vi "19052_get_test_times.vi"(8 "error in (no error)":errorcluster, 9 "modes":string[](array[string]), 10 "steps":u16[](array[numeric]), 11 "VISA Refnum in":refnum<visa-resource-name>) -> (0 "error out":errorcluster, 2 "times":string[](array[string]), 3 "VISA Refnum out":refnum<visa-resource-name>)   [LabVIEW 2015]
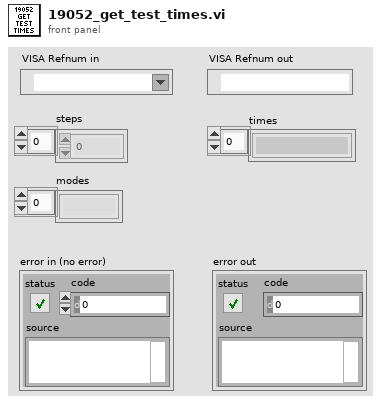
[diagram p1: front panel]
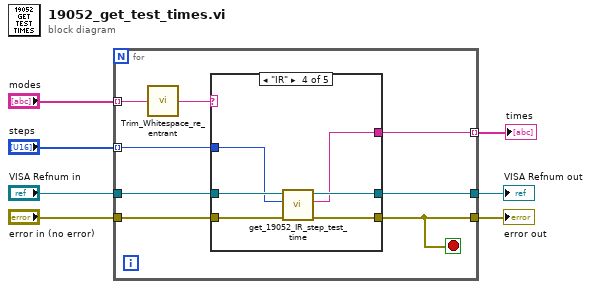
[diagram p0: block diagram]
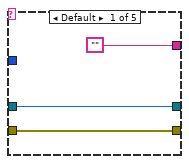
[diagram p2: hidden frame]
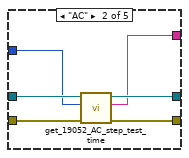
[diagram p3: hidden frame]
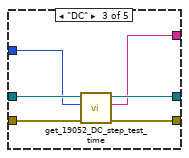
[diagram p4: hidden frame]
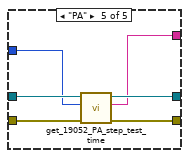
[diagram p5: hidden frame]
diagram:
  n1 = for {
    tunnel: "steps" -> [w15] mode=indexing
    tunnel: "VISA Refnum in" -> [w14]
    tunnel: "error in (no error)" -> [w13]
    tunnel: [w10] -> w5
    tunnel: [w12] -> w6 mode=indexing
    tunnel: [w9] -> w7
    tunnel: "modes" -> [w8] mode=indexing
    stop <- w10 stop-if-true
    n2 = call "Trim_Whitespace_re_entrant.vi"("string"=w8) -> ("trimmed string"=w11:string)  [unwired: 3 in]
    n3 = case shown="\"IR\"" w11 {
      tunnel: w15 -> [_ w23 w27 w33 w39]
      tunnel: w14 -> [w16 w24 w30 w36 w42]
      tunnel: w13 -> [w18 w22 w29 w35 w41]
      tunnel: [w18 w21 w28 w34 w40] -> w10
      tunnel: ["" w19 w25 w31 w37] -> w12
      tunnel: [w16 w20 w26 w32 w38] -> w9
      frame Default {
      }
      frame "AC" {
        n4 = call "get_19052_AC_step_test_time.vi"("error in (no error)"=w22, "Step"=w23, "VISA resource in"=w24) -> ("error out"=w21:errorcluster, "AC total time"=w19:string, "VISA resource out"=w20:refnum<visa-resource-name>)  [unwired: 6 in]
      }
      frame "DC" {
        n5 = call "get_19052_DC_step_test_time.vi"("error in (no error)"=w29, "Step"=w27, "VISA resource in"=w30) -> ("error out"=w28:errorcluster, "DC total time"=w25:string, "VISA resource out"=w26:refnum<visa-resource-name>)  [unwired: 6 in]
      }
      frame "IR" {
        n6 = call "get_19052_IR_step_test_time.vi"("error in (no error)"=w35, "Step"=w33, "VISA resource in"=w36) -> ("error out"=w34:errorcluster, "IR total time"=w31:string, "VISA resource out"=w32:refnum<visa-resource-name>)  [unwired: 6 in]
      }
      frame "PA" {
        n7 = call "get_19052_PA_step_test_time.vi"("error in (no error)"=w41, "step"=w39, "VISA resource in"=w42) -> ("error out"=w40:errorcluster, "PA total time"=w37:string, "VISA resource out"=w38:refnum<visa-resource-name>)  [unwired: 6 in]
      }
    }
  }
  "VISA Refnum out" <- w7
  "times" <- w6
  "error out" <- w5
